vi "CANOpen Channel.vi"(8 "error in (no error)":errorcluster, 11 "Node Ptr":T3 format="%.0x") -> (0 "error out":errorcluster)   [LabVIEW 2021, in "CANOpen Addon System Explorer.lvlib"]
uses:
  CANOpen Addon System Explorer.lvlib
  <vilib>/NI VeriStand/Custom Device API/Custom Device Item Ref.ctl
  Shared/CANOpen_PDO Data Type.ctl
  Shared/CANopen Byte Order.ctl
  Shared/CANOpen Addon GUID Lookup Global.vi
  <vilib>/NI VeriStand/Custom Device API/Get Item Property (Variant).vi
  <vilib>/NI VeriStand/Custom Device API/Set Item Property (Variant).vi
  <vilib>/NI VeriStand/Custom Device API/Custom Device API.lvlib
  Shared/CANOpen Addon Shared.lvlib
panel:
  in  "*Byte Order":T1=enum."little-endian" caption="Byte Order"
  in  "*Bit Offset":u8 caption="Bit Offset" max=8 step=1
  in  "SHDocVw.IWebBrowser2":refnum<k7>(container)
  in  "*Data Type":T2 caption="Data Type"
  in  "*Byte Offset":u8 caption="Byte Offset" max=8 step=1
  in  "*Scale Offset":dbl caption="Scale Offset"
  in  "*Scale Factor":dbl caption="Scale Factor"
  in  "Header":cluster{"Section Name":string}={"Section Name"="TPDO"}
  in  "Description":string
  in  "Parameter Name":string
  # "NI VeriStand channel value = (CANopen received value * Scale Factor) + Scale Offset"
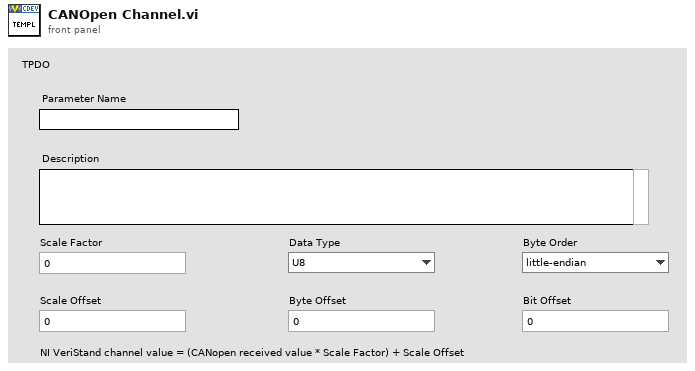
[diagram p1: front panel]
types:
  T1 = typedef "CANOpen Addon Shared.lvlib/CANopen Byte Order.ctl" = enum16{"big-endian network order", "little-endian"}
  T2 = typedef "CANOpen Addon Shared.lvlib/CANOpen_PDO Data Type.ctl" = enum16{"U8", "U16", "U32", "I8", "I16", "I32", "Single", "Double", "Boolean"}
  T3 = typedef "Custom Device API.lvlib/Custom Device Item Ref.ctl" = u64
  T4 = typedef "Custom Device API.lvlib/Custom Device Item Info.ctl" = cluster{"Name":string, "Is Channel":bool, "GUID":string, "Is Waveform":bool}
  T5 = typedef "Custom Device API.lvlib/Custom Device Commands.ctl" = enum16{"Default", "Item renamed", "Shutdown", "Dynamic button pressed"}
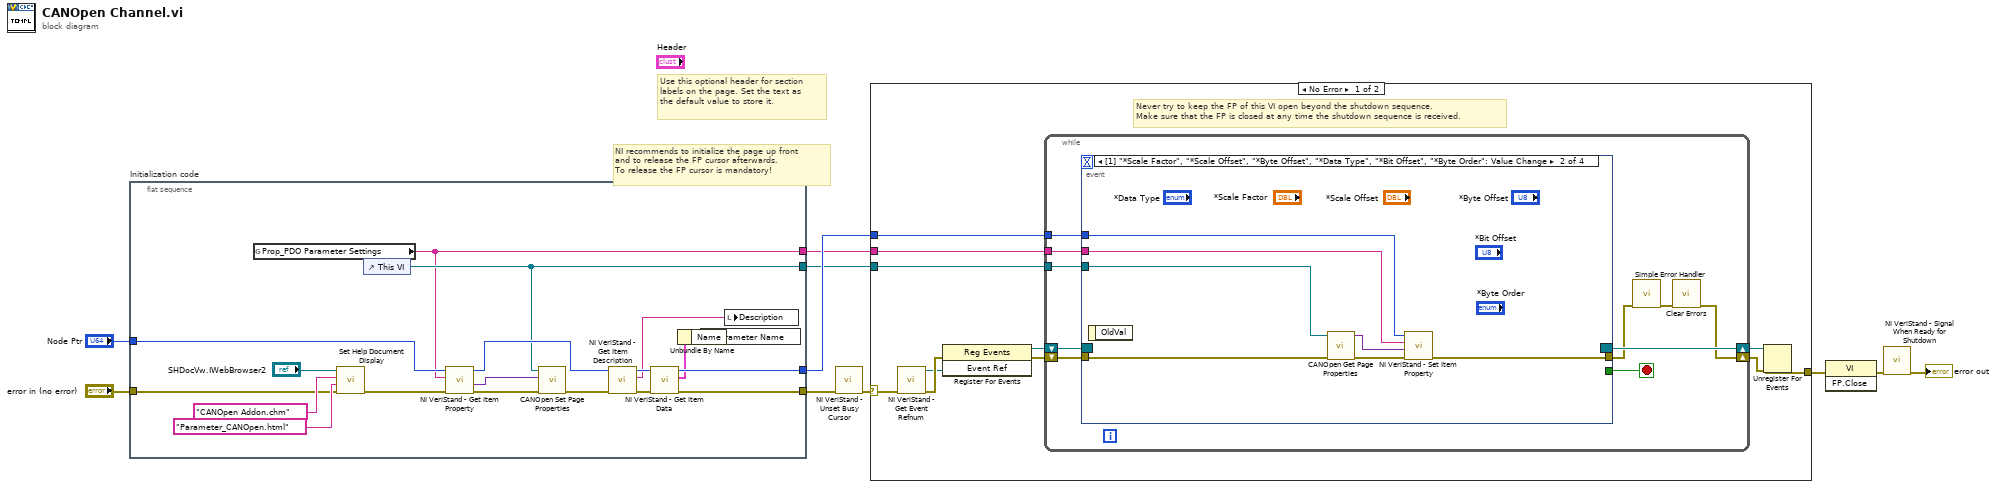
[diagram p0: block diagram]
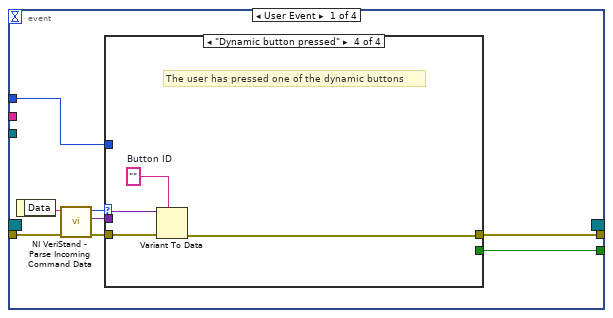
[diagram p2: hidden frame]
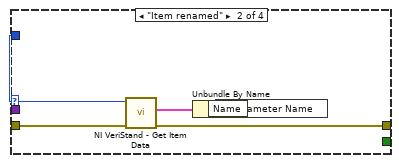
[diagram p4: hidden frame]
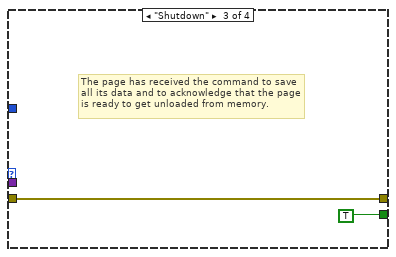
[diagram p5: hidden frame]
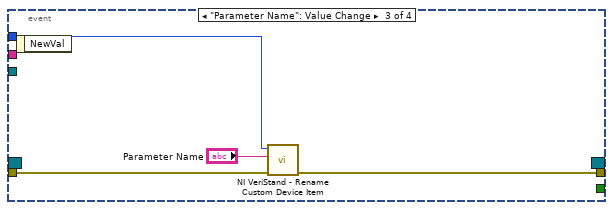
[diagram p6: hidden frame]
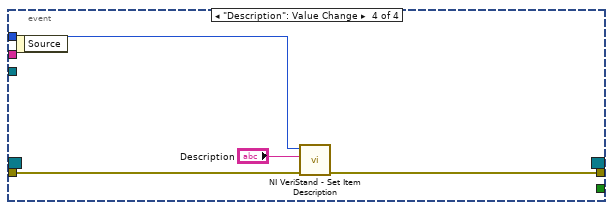
[diagram p7: hidden frame]
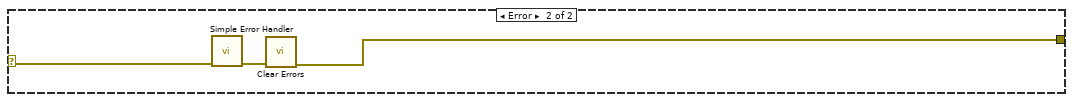
[diagram p8: hidden frame]
diagram:
  # "Use this optional header for section labels on the page. Set the text as the default value to store it."
  # "NI recommends to initialize the page up front\nand to release the FP cursor afterwards.\nTo release the FP cursor is mandatory!"
  n1 = flat-sequence "Initialization code" {
    tunnel: "error in (no error)" -> [w17]
    tunnel: "Node Ptr" -> [w14]
    tunnel: [w23] -> w6
    tunnel: [w29] -> w3
    tunnel: [w12] -> w2
    tunnel: [w11] -> w1
    frame #0 {
      n2 = global read "CANOpen Addon GUID Lookup Global.vi" "Prop_PDO Parameter Settings"() -> (w11:string)
      n3 = call "Set Help Document Display.vi"("error in (no error)"=w17, "HTML File"="Parameter_CANOpen.html", "Main CHM File"="CANOpen Addon.chm", "SHDocVw.IWebBrowser2"="SHDocVw.IWebBrowser2") -> ("error out"=w19:errorcluster)  [unwired: 7 in]
      n4 = control-ref of="This VI"() -> (w12:refnum<vi>)
      n5 = call-poly <vilib>:"NI VeriStand - Get Item Property.vi"("error in (no error)"=w19, "Property Name"=w11, "Item Ref in"=w14) -> ("error out"=w16:errorcluster, "Value"=w18:variant, "Item Ref out"=w13:T3)  [unwired: 5 in, 1 out]
      n6 = call "CANOpen Set Page Properties.vi"("error in"=w16, "variant"=w18, "This VI"=w12) -> ("error out"=w15:errorcluster)  [unwired: 8 in]
      n7 = call <vilib>:"NI VeriStand - Get Item Description.vi"("error in (no error)"=w15, "Item Ref in"=w13) -> ("error out"=w26:errorcluster, "Description"=w27:string, "Item Ref out"=w28:T3)  [unwired: 7 out]
      n8 = call <vilib>:"NI VeriStand - Get Item Data.vi"("error in (no error)"=w26, "Item Ref in"=w28) -> ("error out"=w23:errorcluster, "Item Info"=w25:T4, "Item Ref out"=w29:T3)  [unwired: 7 out]
      n9 = Unbundle By Name(w25) -> ("Name"=w24:string)
      n10 = local write "Parameter Name"(w24) -> ()
      n11 = local write "Description"(w27) -> ()
    }
  }
  n12 = call <vilib>:"NI VeriStand - Unset Busy Cursor.vi"("error in (no error)"=w6) -> ("error out"=w5:errorcluster)  [unwired: 10 out]
  n13 = case shown="No Error" w5 {
    selector: w5 -> [w32 w88]
    tunnel: [w37 w86] -> w10
    tunnel: w3 -> [w33 _]
    tunnel: w2 -> [w31 _]
    tunnel: w1 -> [w30 _]
    frame No Error {
      # "Never try to keep the FP of this VI open beyond the shutdown sequence.\nMake sure that the FP is closed at any time the shutdown sequence is received."
      n14 = call <vilib>:"NI VeriStand - Get Event Refnum.vi"("error in (no error)"=w32) -> ("error out"=w40:errorcluster, "Event Ref"=w36:refnum<user-event>)  [unwired: 9 out]
      n15 = register-events(error in=w40, w36) -> (reference out=w34:refnum<event-registration>, error out=w35:errorcluster)  [unwired: 1 in]
      n16 = while {
        tunnel: w33 -> [w46]
        shift-right: [w43] -> w38
        shift-left: w35 -> [w49]
        shift-right: [w50] -> w39
        shift-left: w34 -> [w48]
        tunnel: w31 -> [w42]
        tunnel: w30 -> [w41]
        stop <- w47 stop-if-true
        n17 = event shown="[1] \"*Scale Factor\", \"*Scale Offset\", \"*Byte Offset\", \"*Data Type\", \"*Bit Offset\", \"*Byte Order\": Value Change" {
          selector: w48 -> [_ _ _ _]
          dyn-events: [_ _ _ _] -> w50
          timeout: _ -> [_ _ _ _]
          tunnel: w49 -> [w58 w77 w81 w84]
          tunnel: [w54 _ _ _] -> w47
          tunnel: [w53 w74 w80 w83] -> w45
          tunnel: w46 -> [w52 w72 w79 w85]
          tunnel: w42 -> [_ w76 _ _]
          tunnel: w41 -> [_ w71 _ _]
          event User Event {
            n18 = event-data() -> ("Data"=w57:string)  [unwired: 1 out]
            n19 = call <vilib>:"NI VeriStand - Parse Incoming Command Data.vi"("error in (no error)"=w58, "Incoming data"=w57) -> ("error out"=w56:errorcluster, "Outgoing data"=w51:variant, "Action"=w55:T5)  [unwired: 7 out]
            n20 = case shown="\"Dynamic button pressed\"" w55 {
              tunnel: w56 -> [w59 w64 w65 w70]
              tunnel: [_ _ TRUE _] -> w54
              tunnel: [w59 w61 w65 w67] -> w53
              tunnel: w52 -> [_ w63 _ _]
              tunnel: w51 -> [_ _ _ w69]
              frame "Default", Default {
              }
              frame "Item renamed" {
                n21 = call <vilib>:"NI VeriStand - Get Item Data.vi"("error in (no error)"=w64, "Item Ref in"=w63) -> ("error out"=w61:errorcluster, "Item Info"=w62:T4)  [unwired: 8 out]
                n22 = Unbundle By Name(w62) -> ("Name"=w60:string)
                n23 = local write "Parameter Name"(w60) -> ()
              }
              frame "Shutdown" {
                # "The page has received the command to save all its data and to acknowledge that the page is ready to get unloaded from memory."
              }
              frame "Dynamic button pressed" {
                w68 = ""  # Button ID
                # "The user has pressed one of the dynamic buttons"
                n24 = Variant To Data(error in=w70, type=w68, Variant=w69) -> (error out=w67:errorcluster)  [unwired: 1 out]
              }
            }
          }
          event "*Scale Factor", "*Scale Offset", "*Byte Offset", "*Bit Offset": Value Change {
            n25 = event-data() -> ()  [unwired: 2 out]
            n26 = call "CANOpen Get Page Properties.vi"("error in (no error)"=w77, "This VI"=w76) -> ("error out"=w75:errorcluster, "Settings"=w73:variant)  [unwired: 8 in]
            n27 = call-poly <vilib>:"NI VeriStand - Set Item Property.vi"("error in (no error)"=w75, "Value"=w73, "Property Name"=w71, "Item Ref in"=w72) -> ("error out"=w74:errorcluster)  [unwired: 5 in, 2 out]
          }
          event "Parameter Name": Value Change {
            n28 = event-data() -> ()  [unwired: 2 out]
            n29 = call <vilib>:"NI VeriStand - Rename Custom Device Item.vi"("error in (no error)"=w81, "New Name"="Parameter Name", "Item Ref in"=w79) -> ("error out"=w80:errorcluster)  [unwired: 1 in, 7 out]
          }
          event "Description": Value Change {
            n30 = event-data() -> ()  [unwired: 2 out]
            n31 = call <vilib>:"NI VeriStand - Set Item Description.vi"("error in (no error)"=w84, "Description"="Description", "Item Ref in"=w85) -> ("error out"=w83:errorcluster)  [unwired: 8 out]
          }
        }
        n32 = call <vilib>:"Simple Error Handler.vi"("error in (no error)"=w45) -> ("error out"=w44:errorcluster)  [unwired: 1 in, 7 out]
        n33 = call <vilib>:"Clear Errors.vi"("error in (no error)"=w44) -> ("error out"=w43:errorcluster)  [unwired: 1 in, 5 out]
      }
      n34 = Unregister For Events(event registration refnum=w39, error in=w38) -> (error out=w37:errorcluster)
    }
    frame Error {
      n35 = call <vilib>:"Simple Error Handler.vi"("error in (no error)"=w88) -> ("error out"=w87:errorcluster)  [unwired: 1 in, 7 out]
      n36 = call <vilib>:"Clear Errors.vi"("error in (no error)"=w87) -> ("error out"=w86:errorcluster)  [unwired: 1 in, 5 out]
    }
  }
  n37 = invoke class="VI" method="FP.Close"(error in=w10) -> (error out=w9:errorcluster)  [unwired: 2 in, 2 out]
  n38 = call <vilib>:"NI VeriStand - Signal When Ready for Shutdown.vi"("error in (no error)"=w9) -> ("error out"=→"error out":errorcluster)  [unwired: 10 out]
